vi "Load Simulation.vi"(0 "reference in":refnum<class "Battery.lvclass">, 2 "Simulation Parameters":T1={"num_rc_pairs"=1, "R0"=0.0015, "R1"=0.001, "C1"=2500.0, "R2"=0.0008, "C2"=40000.0, " nominal_capacity_Ah"=5.0, "upper_voltage_cutoff"=4.2, "lower_voltage_cutoff"=3.0} {"lower_voltage_cutoff" format="%#_13g"; "upper_voltage_cutoff" format="%#_13g"; "nominal_capacity_Ah" format="%#_13g"; "C2" format="%#_13g"; "R2" format="%#_13g"; "C1" format="%#_13g"; "R1" format="%#_13g"; "R0" format="%#_13g"}, 5 "Error In":errorcluster) -> (14 "reference out":refnum<class "Battery.lvclass">, 16 "simulation loaded":bool, 19 "Error Out":errorcluster)   [LabVIEW 2023, in "Battery.lvclass"]
uses:
  Battery.lvclass
  Simulation Parameters.ctl
  Battery.lvclass/Battery.ctl
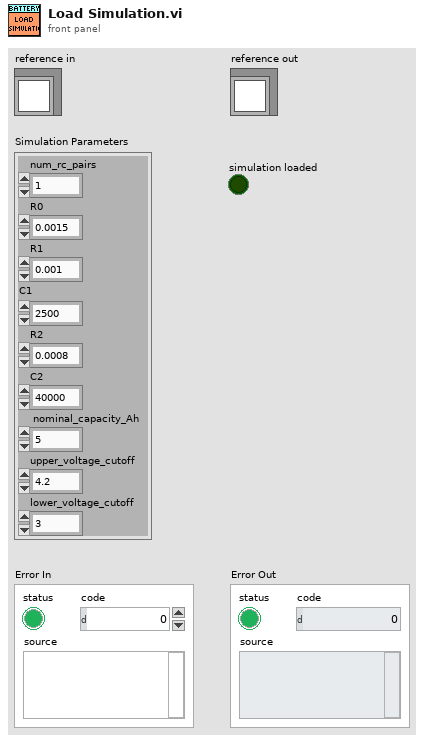
[diagram p1: front panel]
types:
  T1 = typedef "Battery.lvclass/Simulation Parameters.ctl" = cluster{"num_rc_pairs":i32, "R0":dbl, "R1":dbl, "C1":dbl, "R2":dbl, "C2":dbl, " nominal_capacity_Ah":dbl, "upper_voltage_cutoff":dbl, "lower_voltage_cutoff":dbl}
  T2 = typedef "Battery.lvclass/ObjectAttributes.ctl" = cluster{"Python module":path, "Python Session":refnum<k35>, "PybammWrapper":refnum<k38>, "model loaded":bool, "simulation loaded":bool, "simulation enabled":bool, "SOC OCV Curve":dbl[][], "Open Circuit Voltage (V)":dbl, "State of Charge (%)":dbl, "HPS17K Refs":refnum<class "HPS-17000.lvclass">[], "# Cells in Series":u16, "# Cells in Parallel":u16, "Model Parameters":T3, "Simulation Parameters":T1}
  T3 = typedef "Battery.lvclass/Model Parameters.ctl" = cluster{"chemistry":string, "model_type":string}
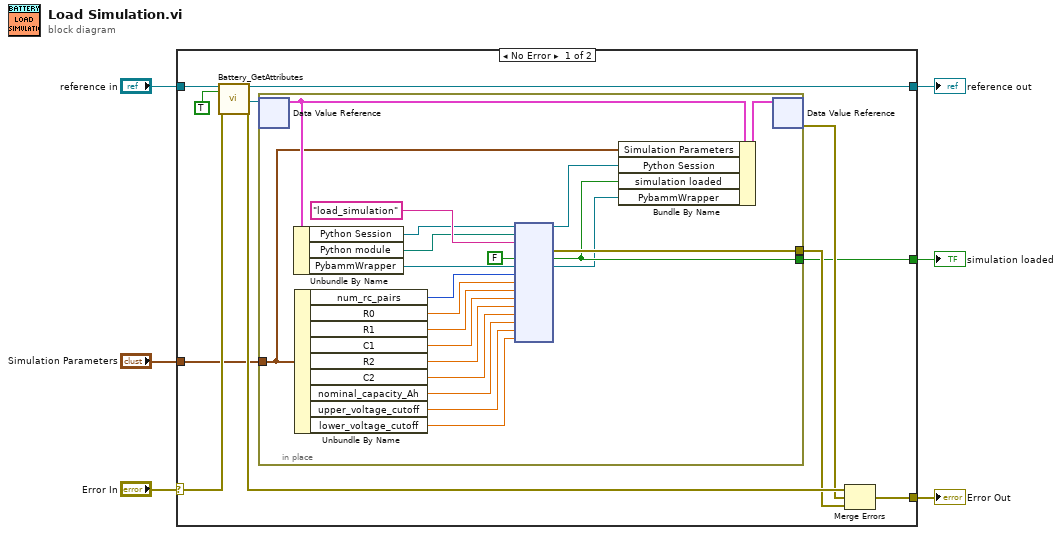
[diagram p0: block diagram]
diagram:
  n1 = case shown="No Error" "Error In" {
    selector: "Error In" -> [w16 w40]
    tunnel: [w14 w40] -> w5
    tunnel: [w15 w39] -> w3
    tunnel: "reference in" -> [w17 w39]
    tunnel: "Simulation Parameters" -> [w9 _]
    tunnel: [w7 _] -> w1
    frame No Error {
      n2 = call "Battery_GetAttributes.vi"("reference in"=w17, "OnlyGetDvrReference(False)"=TRUE, "Error In"=w16) -> ("reference out"=w15:refnum<class "Battery.lvclass">, "DataRef"=w13:refnum<data-value>, "Error Out"=w11:errorcluster)  [unwired: 13 in, 1 out]
      n3 = in-place {
        in-place-border: w9 -> [w18]
        in-place-border: [w25] -> w8
        in-place-border: [w24] -> w7
        n4 = in-place-dvr #1(w13) -> (w37:T2)  [unwired: 1 out]
        n5 = Unbundle By Name(w37) -> ("Python Session"=w21:refnum<k35>, "Python module"=w22:path, "PybammWrapper"=w23:refnum<k38>)
        n6 = Unbundle By Name(w18) -> ("num_rc_pairs"=w34:i32, "R0"=w33:dbl, "R1"=w32:dbl, "C1"=w31:dbl, "R2"=w30:dbl, "C2"=w29:dbl, "nominal_capacity_Ah"=w28:dbl, "upper_voltage_cutoff"=w27:dbl, "lower_voltage_cutoff"=w26:dbl)
        n7 = node(w21, w22, "load_simulation" ("function name"), FALSE, w23, w34, w33, w32, w31, w30, w29, w28, w27, w26) -> (w20:refnum<k35>, w25:errorcluster, w24:bool, w19:refnum<k38>)  [unwired: 10 in, 2 out]
        n8 = Bundle By Name(cluster=w37, "Simulation Parameters"=w18, "Python Session"=w20, "simulation loaded"=w24, "PybammWrapper"=w19) -> (w38:T2)
        n9 = in-place-dvr #1(w38) -> (w10:errorcluster)  [unwired: 1 out]
      }
      n10 = Merge Errors(w11, w10, w8) -> (w14:errorcluster)
    }
    frame Error {
    }
  }
  "Error Out" <- w5
  "reference out" <- w3
  "simulation loaded" <- w1
